vi "Escrita TDMS.vi"() -> ()   [LabVIEW 2018]
panel:
  in  "stop":bool
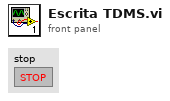
[diagram p1: front panel]
types:
  T1 = enum16{"open", "open or create", "create or replace", "create", "open (read-only)"}
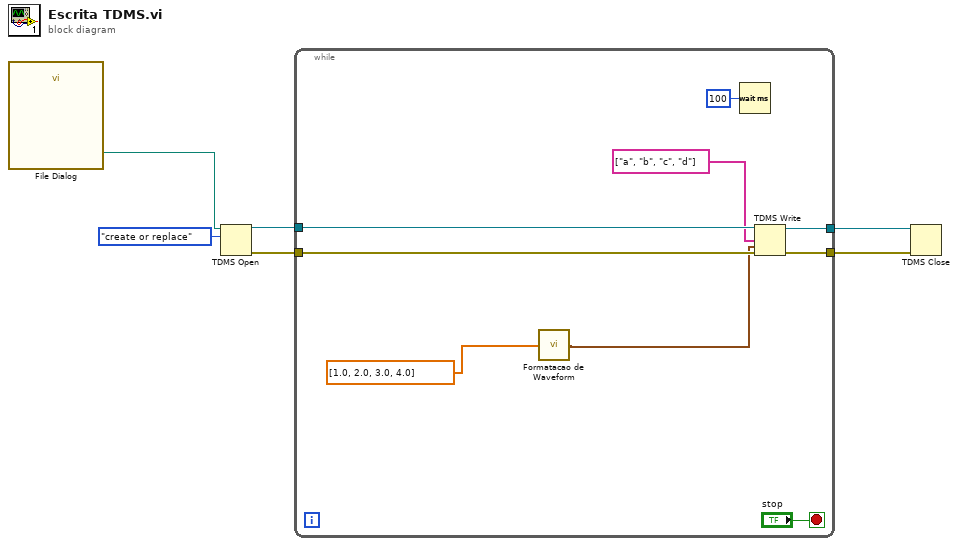
[diagram p0: block diagram]
diagram:
  n1 = call "File Dialog"() -> ("selected path"=w1:path)  [unwired: 12 in, 3 out]
  n2 = TDMS Open(10:T1."create or replace" ("operation (0:open)"), 11:w1) -> (0:w5:errorcluster, 3:w6:refnum<k34>)  [unwired: 5 in]
  n3 = while {
    tunnel: w6 -> [w15]
    tunnel: w5 -> [w14]
    tunnel: [w13] -> w4
    tunnel: [w12] -> w3
    stop <- "stop" stop-if-true
    n4 = call "Formatacao de Waveform.vi"("Array in"=dbl[] [1.0, 2.0, 3.0, 4.0]) -> ("Array out"=w8:waveform(dbl)[])  [unwired: 2 in]
    n5 = Wait (ms)(milliseconds to wait=u32 100) -> ()  [unwired: 1 out]
    n6 = TDMS Write(0:w15, 7:string[] ["a", "b", "c", "d"], 9:w8, 11:w14) -> (4:w13:refnum<k34>, 15:w12:errorcluster)  [unwired: 2 in, 2 out]
  }
  n7 = TDMS Close(8:w3, 11:w4) -> ()  [unwired: 2 out]
